vi "Destroy.vi"(0 "reference in":refnum<class "DemoClass1.lvclass">, 5 "error in (no error)":errorcluster) -> (14 "reference out":refnum<class "DemoClass1.lvclass">, 19 "error out":errorcluster)   [LabVIEW 2017, in "DemoClass1.lvclass"]
uses:
  DemoClass1.lvclass
  C:/Program Files/National Instruments/LabVIEW 2017/vi.lib/addons/_AddQ/G#Object/G#Object.lvclass
  <vilib>/addons/_AddQ/G#Object/G#Object.lvclass
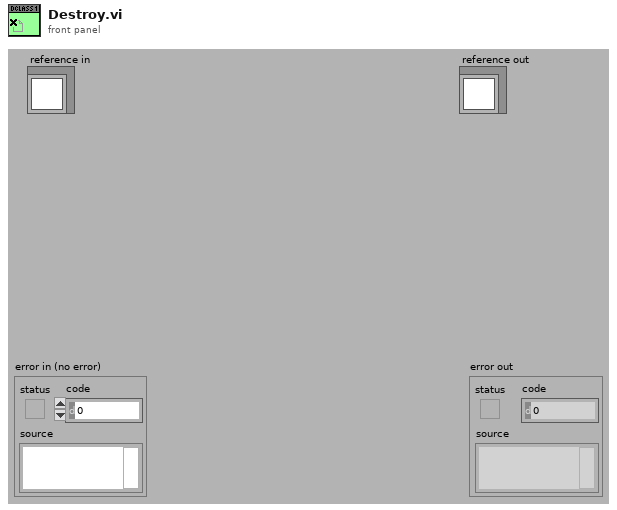
[diagram p1: front panel]
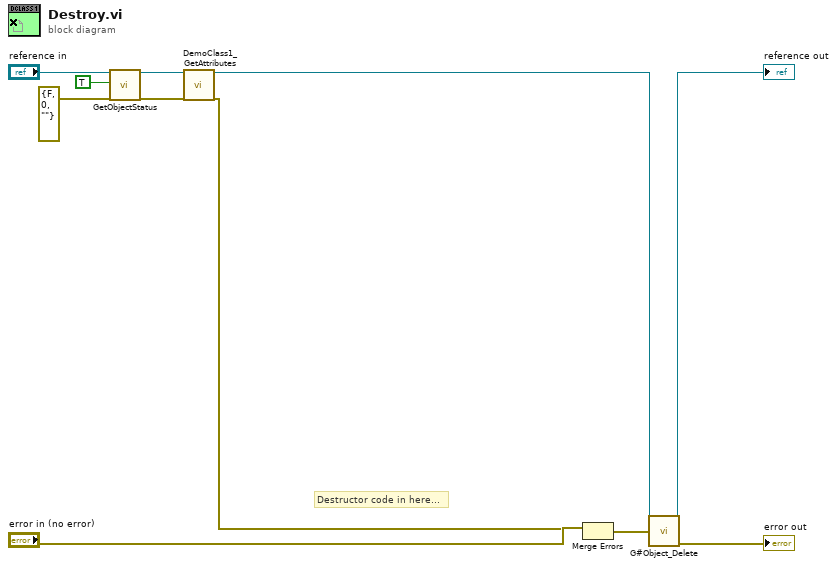
[diagram p0: block diagram]
diagram:
  # "Destructor code in here..."
  n1 = call-dynamic "GetObjectStatus.vi"("reference in"="reference in", "simple info (F)"=TRUE ("Simple Info"), "error in (no error)"=errorcluster {"status"=FALSE, "code"=0, "source"=""}) -> ("reference out"=w5:refnum<class "DemoClass1.lvclass">, "error out"=w2:errorcluster)  [unwired: 5 in, 10 out]
  n2 = call "DemoClass1_GetAttributes.vi"("reference in"=w5, "error in (no error)"=w2) -> ("reference out"=w9:refnum<class "DemoClass1.lvclass">, "error out"=w7:errorcluster)  [unwired: 1 in, 15 out]
  n3 = Merge Errors("error in (no error)", w7) -> (w8:errorcluster)
  n4 = call <vilib>:"G#Object_Delete.vi"("reference in"=w9, "error in (no error)"=w8) -> ("reference out"=→"reference out":refnum<class "DemoClass1.lvclass">, "error out"=→"error out":errorcluster)  [unwired: 16 in]
